vi "CameraTest.vi"() -> ()   [LabVIEW 2016]
uses:
  <vilib>/userdefined/High Color/IMAQdx.ctl
  ListboxMenu/listbox/listbox.lvclass
  ListboxMenu/listbox/listbox.lvclass/listbox.ctl
  ListboxMenu/LNK/UP/UP.lvclass
  C:/Users/ok/Desktop/camera parameters/ListboxMenu/LNK/Parent Class/Menu.lvclass
  ListboxMenu/LNK/Delete/Delete.lvclass
  ListboxMenu/LNK/Down/Down.lvclass
  <vilib>/Utility/miscctls.llb/LVRowAndColumnTypeDef.ctl
  <vilib>/Utility/miscctls.llb/LVPositionTypeDef.ctl
  <vilib>/vision/driver/NI_Vision_Acquisition_Software.lvlib
  <resource>/objmgr/imaqdx.rc
  <vilib>/ptbypt/NI_PtbyPt.lvlib
panel:
  in  "搜索相机":bool
  in  "启动相机":bool
  in  "停止相机":bool
  in  "连续获取":bool
  in  "单次获取":bool
  out "Image":T1(plugin-control)
  in  "Enum":u16(ring) items=["Off", "On"]
  in  "String":string
  in  "U32":i16
  in  "I64":i64
  in  "DBL":dbl
  in  "Bool":bool
  in  "写入参数文件":bool
  in  "读取参数文件":bool
  in  "相机参数列表":u16(ring) items=["NULL", "AcquisitionAttributes::AdvancedEthernet::BandwidthControl::DesiredPeakBandwidth", "AcquisitionAttributes::AdvancedEthernet::Controller::DestinationMode", "AcquisitionAttributes::AdvancedEthernet::Controller::DestinationMulticastAddress", "AcquisitionAttributes::AdvancedEthernet::EventParameters::MaxOutstandingEvents", "AcquisitionAttributes::AdvancedEthernet::FirewallTraversal::Enabled", "AcquisitionAttributes::AdvancedEthernet::FirewallTraversal::KeepAliveTime", "AcquisitionAttributes::AdvancedEthernet::ResendParameters::MaxResendsPerPacket", "AcquisitionAttributes::AdvancedEthernet::ResendParameters::MemoryWindowSize", "AcquisitionAttributes::AdvancedEthernet::ResendParameters::MissingPacketTimeout", "AcquisitionAttributes::AdvancedEthernet::ResendParameters::NewPacketTimeout", "AcquisitionAttributes::AdvancedEthernet::ResendParameters::ResendBatchingPercentage", "AcquisitionAttributes::AdvancedEthernet::ResendParameters::ResendResponseTimeout", "AcquisitionAttributes::AdvancedEthernet::ResendParameters::ResendThresholdPercentage", "AcquisitionAttributes::AdvancedEthernet::ResendParameters::ResendTimerResolution", "AcquisitionAttributes::AdvancedEthernet::ResendParameters::ResendsEnabled", "AcquisitionAttributes::AdvancedEthernet::TestPacketParameters::MaxTestPacketRetries", "AcquisitionAttributes::AdvancedEthernet::TestPacketParameters::TestPacketEnabled", "AcquisitionAttributes::AdvancedEthernet::TestPacketParameters::TestPacketTimeout", "AcquisitionAttributes::AdvancedGenicam::CommandTimeout", "AcquisitionAttributes::AdvancedGenicam::EventsEnabled", "AcquisitionAttributes::AdvancedGenicam::IgnoreCameraValidationErrors", "AcquisitionAttributes::Bayer::Algorithm", "AcquisitionAttributes::Bayer::GainB", "AcquisitionAttributes::Bayer::GainG", "AcquisitionAttributes::Bayer::GainR", "AcquisitionAttributes::Bayer::Pattern", "AcquisitionAttributes::ChunkDataDecoding::ChunkDataDecodingEnabled", "AcquisitionAttributes::ChunkDataDecoding::MaximumChunkCopySize", "CameraAttributes::AnalogControls::GainAuto", "CameraAttributes::AnalogControls::GainSelector", "CameraAttributes::AnalogControls::GainRaw", "CameraAttributes::AnalogControls::BlackLevelSelector", "CameraAttributes::AnalogControls::BlackLevelRaw", "CameraAttributes::AnalogControls::GammaEnable", "CameraAttributes::AnalogControls::GammaSelector", "CameraAttributes::AnalogControls::Gamma", "CameraAttributes::AnalogControls::DigitalShift", "CameraAttributes::ImageFormat::PixelFormat", "CameraAttributes::ImageFormat::ReverseX", "CameraAttributes::ImageFormat::TestImageSelector", "CameraAttributes::AOI::Width", "CameraAttributes::AOI::Height", "CameraAttributes::AOI::OffsetX", "CameraAttributes::AOI::OffsetY", "CameraAttributes::AOI::CenterX", "CameraAttributes::AOI::CenterY", "CameraAttributes::AOI::BinningHorizontal", "CameraAttributes::AOI::BinningVertical", "CameraAttributes::AcquisitionTrigger::AcquisitionMode", "CameraAttributes::AcquisitionTrigger::AcquisitionFrameCount", "CameraAttributes::AcquisitionTrigger::TriggerSelector", "CameraAttributes::AcquisitionTrigger::TriggerMode", "CameraAttributes::AcquisitionTrigger::TriggerSoftware", "CameraAttributes::AcquisitionTrigger::TriggerSource", "CameraAttributes::AcquisitionTrigger::TriggerActivation", "CameraAttributes::AcquisitionTrigger::TriggerDelayAbs", "CameraAttributes::AcquisitionTrigger::ExposureMode", "CameraAttributes::AcquisitionTrigger::ExposureAuto", "CameraAttributes::AcquisitionTrigger::ExposureTimeAbs", "CameraAttributes::AcquisitionTrigger::ExposureTimeRaw", "CameraAttributes::AcquisitionTrigger::GlobalResetReleaseModeEnable", "CameraAttributes::AcquisitionTrigger::AcquisitionFrameRateEnable", "CameraAttributes::AcquisitionTrigger::AcquisitionFrameRateAbs", "CameraAttributes::AcquisitionTrigger::AcquisitionStatusSelector", "CameraAttributes::DigitalIO::LineSelector", "CameraAttributes::DigitalIO::LineMode", "CameraAttributes::DigitalIO::LineFormat", "CameraAttributes::DigitalIO::LineSource", "CameraAttributes::DigitalIO::LineInverter", "CameraAttributes::DigitalIO::UserOutputSelector", "CameraAttributes::DigitalIO::UserOutputValue", "CameraAttributes::DigitalIO::UserOutputValueAll", "CameraAttributes::SequenceControl::SequenceEnable", "CameraAttributes::SequenceControl::SequenceControlConfiguration::SequenceAdvanceMode", "CameraAttributes::SequenceControl::SequenceSetTotalNumber", "CameraAttributes::SequenceControl::SequenceSetIndex", "CameraAttributes::SequenceControl::SequenceSetStore", "CameraAttributes::SequenceControl::SequenceSetLoad", "CameraAttributes::SequenceControl::SequenceSetExecutions", "CameraAttributes::TimerControls::TimerDelayTimebaseAbs", "CameraAttributes::TimerControls::TimerDurationTimebaseAbs", "CameraAttributes::TimerControls::TimerSelector", "CameraAttributes::TimerControls::TimerDelayAbs", "CameraAttributes::TimerControls::TimerDelayRaw", "CameraAttributes::TimerControls::TimerDurationAbs", "CameraAttributes::TimerControls::TimerDurationRaw", "CameraAttributes::TimerControls::TimerTriggerSource", "CameraAttributes::TimerControls::TimerTriggerActivation", "CameraAttributes::TimerControls::CounterSelector", "CameraAttributes::TimerControls::CounterEventSource", "CameraAttributes::TimerControls::CounterResetSource", "CameraAttributes::LUTControls::LUTSelector", "CameraAttributes::LUTControls::LUTEnable", "CameraAttributes::LUTControls::LUTIndex", "CameraAttributes::LUTControls::LUTValue", "CameraAttributes::UserDefinedValues::UserDefinedValueSelector", "CameraAttributes::UserDefinedValues::UserDefinedValue", "CameraAttributes::DeviceInformation::DeviceUserID", "CameraAttributes::ChunkDataStreams::ChunkModeActive", "CameraAttributes::EventsGeneration::EventSelector", "CameraAttributes::EventsGeneration::EventNotification", "CameraAttributes::UserSets::UserSetSelector", "CameraAttributes::UserSets::UserSetLoad", "CameraAttributes::UserSets::UserSetSave", "CameraAttributes::UserSets::UserSetDefaultSelector", "CameraAttributes::UserSets::DefaultSetSelector", "CameraAttributes::TransportLayer::GevSCFTD", "CameraAttributes::TransportLayer::GevSCBWR", "CameraAttributes::TransportLayer::GevSCBWRA", "CameraAttributes::TransportLayer::GevTimestampControlReset", "CameraAttributes::TransportLayer::GevTimestampControlLatchReset", "CameraAttributes::FileAccessControl::FileSelector", "CameraAttributes::FileAccessControl::FileOperationSelector", "CameraAttributes::FileAccessControl::FileOpenMode", "CameraAttributes::FileAccessControl::FileAccessOffset", "CameraAttributes::FileAccessControl::FileAccessLength", "CameraAttributes::FileAccessControl::FileOperationExecute", "CameraAttributes::AutoFunctions::AutoTargetValue", "CameraAttributes::AutoFunctions::AutoGainRawLowerLimit", "CameraAttributes::AutoFunctions::AutoGainRawUpperLimit", "CameraAttributes::AutoFunctions::AutoExposureTimeAbsLowerLimit", "CameraAttributes::AutoFunctions::AutoExposureTimeAbsUpperLimit", "CameraAttributes::AutoFunctions::AutoFunctionProfile", "CameraAttributes::AutoFunctions::AutoFunctionAOIs::AutoFunctionAOISelector", "CameraAttributes::AutoFunctions::AutoFunctionAOIs::AutoFunctionAOIWidth", "CameraAttributes::AutoFunctions::AutoFunctionAOIs::AutoFunctionAOIHeight", "CameraAttributes::AutoFunctions::AutoFunctionAOIs::AutoFunctionAOIOffsetX", "CameraAttributes::AutoFunctions::AutoFunctionAOIs::AutoFunctionAOIOffsetY", "CameraAttributes::AutoFunctions::AutoFunctionAOIs::AutoFunctionAOIUsageIntensity", "CameraAttributes::AutoFunctions::AutoFunctionAOIs::AutoFunctionAOIUsageWhiteBalance", "CameraAttributes::ExpertFeatureAccess::ExpertFeatureAccessSelector", "CameraAttributes::ExpertFeatureAccess::ExpertFeatureAccessKey", "AcquisitionAttributes::BitsPerPixel", "AcquisitionAttributes::ImageDecoderCopyMode", "AcquisitionAttributes::IncompleteBufferMode", "AcquisitionAttributes::OutputImageType", "AcquisitionAttributes::OverwriteMode", "AcquisitionAttributes::PacketSize", "AcquisitionAttributes::ReceiveTimestampMode", "AcquisitionAttributes::ShiftPixelBits", "AcquisitionAttributes::SwapPixelBytes", "AcquisitionAttributes::Timeout"]
  in  "添加参数":bool
  in  "写入参数":bool
  in  "获取参数值":bool
  in  "打开相机":bool
  in  "相机参数":i32(listbox)
  in  "相机列表":u16(ring) items=["acA2500-14gm:\"cam0\""]
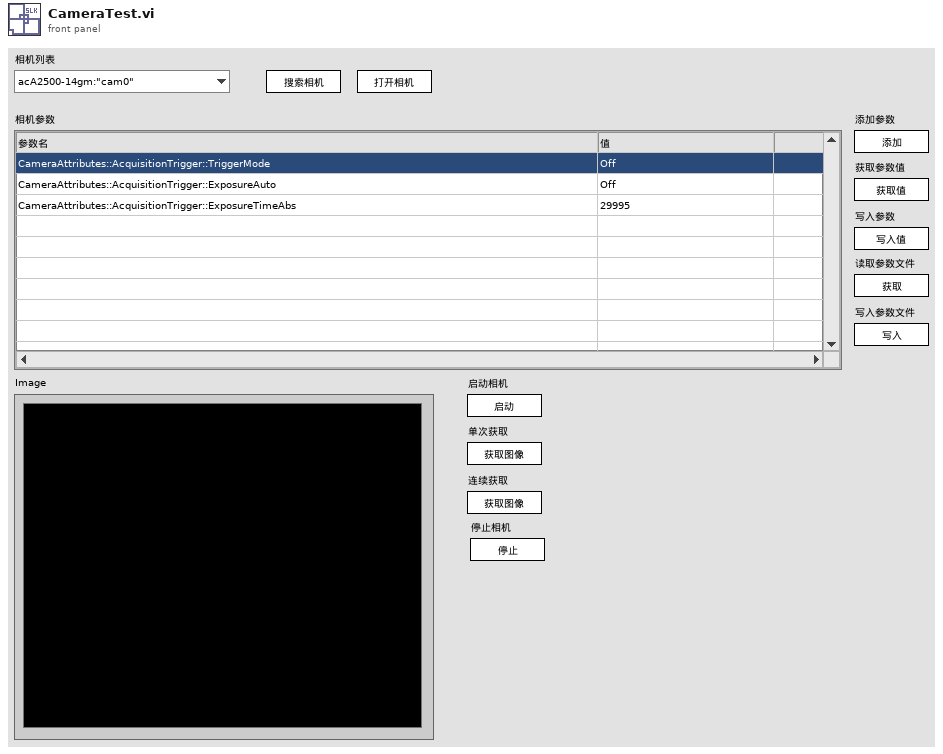
[diagram p1: front panel]
types:
  T1 = typedef "IMAQ Image.ctl" = refnum<image>
  T2 = typedef "Image Type" = u32
  T3 = typedef "IMAQdx.ctl" = refnum<k21>
  T4 = typedef "LVRowAndColumnTypeDef.ctl" = cluster{"Row":i32, "Column":i32}
  T5 = typedef "LVPositionTypeDef.ctl" = cluster{"Left":i32, "Top":i32}
  T6 = cluster{"Type":u32, "Version":u32, "Flags":u32, "SerialNumberHigh":u32, "SerialNumberLow":u32, "BusType":u32, "InterfaceName":string, "VendorName":string, "ModelName":string, "CameraFileName":string, "CameraAttributeURL":string}[]
  T7 = cluster{"Type":u32, "Version":u32, "Flags":u32, "SerialNumberHigh":u32, "SerialNumberLow":u32, "BusType":u32, "InterfaceName":string, "VendorName":string, "ModelName":string, "CameraFileName":string, "CameraAttributeURL":string}
  T8 = typedef "LVPoint32TypeDef.ctl" = cluster{"Horizontal":i32, "Vertical":i32}
  T9 = typedef "NI_Vision_Acquisition_Software.lvlib/IMAQdx Attribute Type.ctl" = enum32{"U32", "I64", "DBL", "String", "Enum", "Bool", "Command"}
  T10 = cluster{"Attribute Type":T9, "Readable":bool, "Writable":bool, "Attribute Name":string}[]
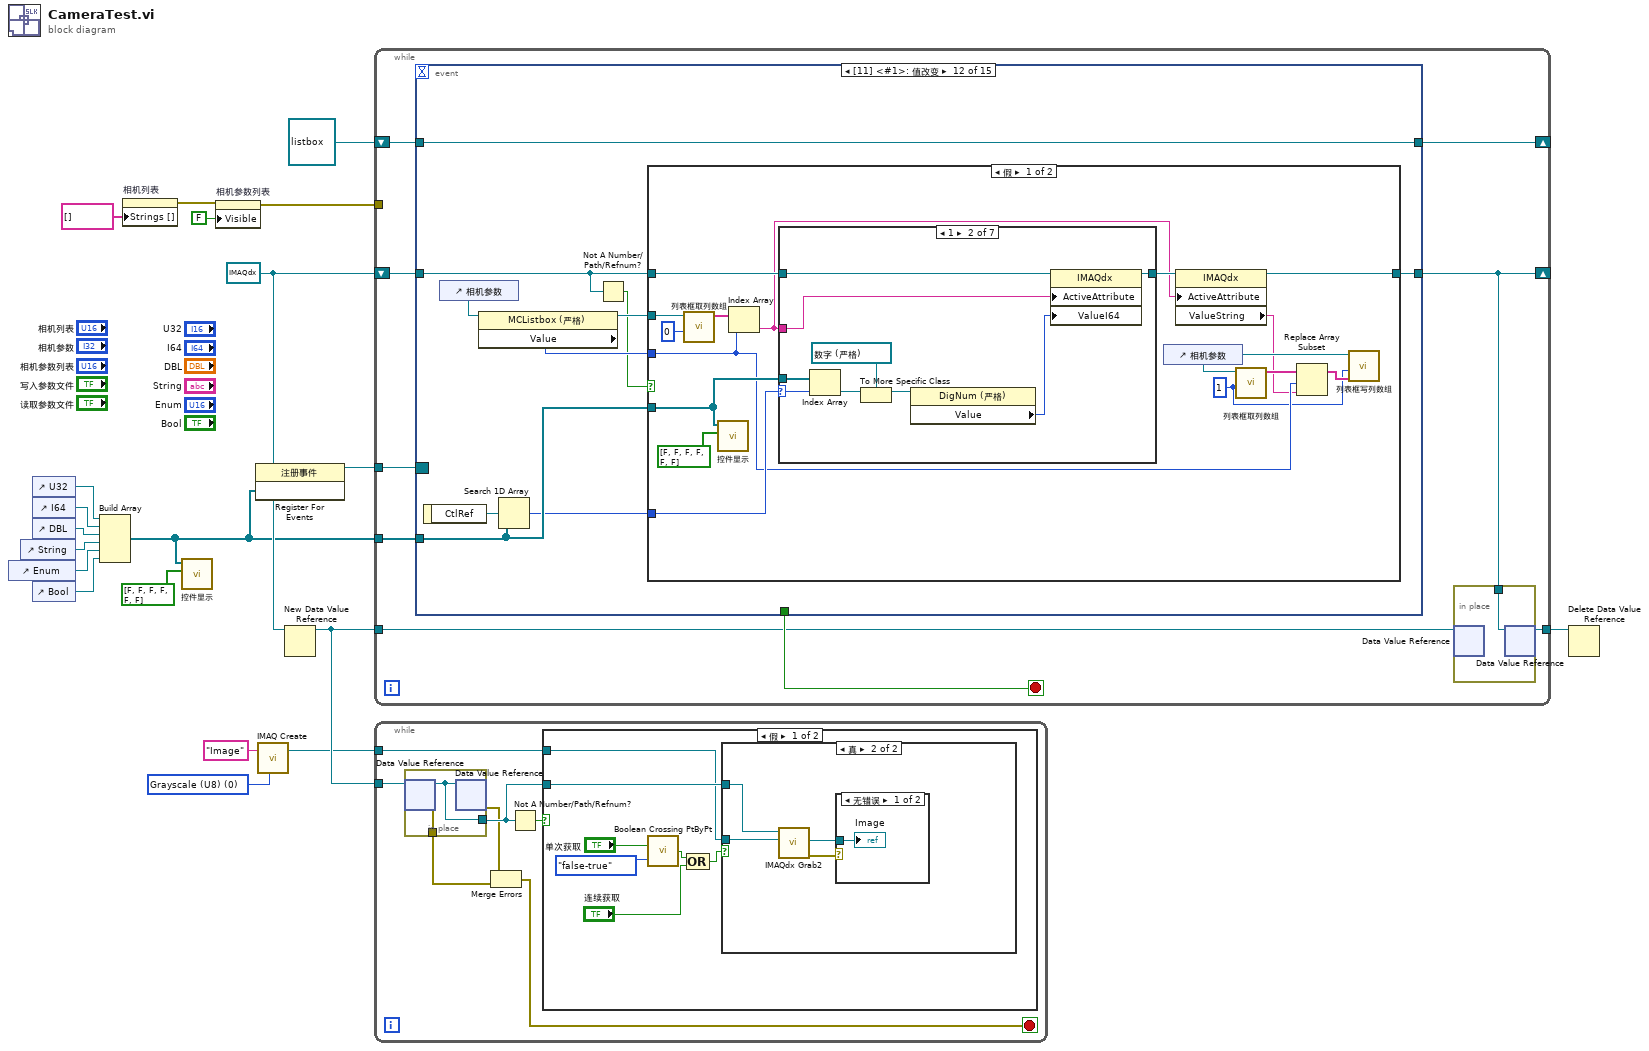
[diagram p0: block diagram]
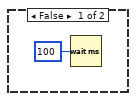
[diagram p2: hidden frame]
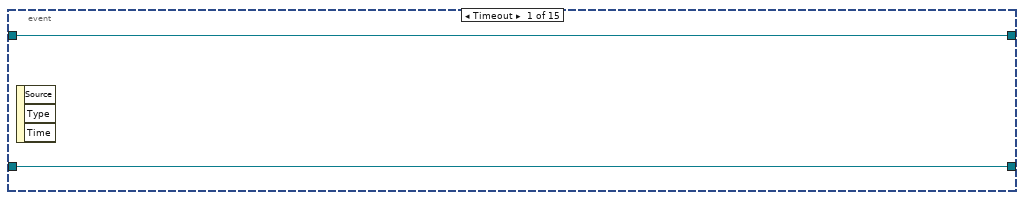
[diagram p5: hidden frame]
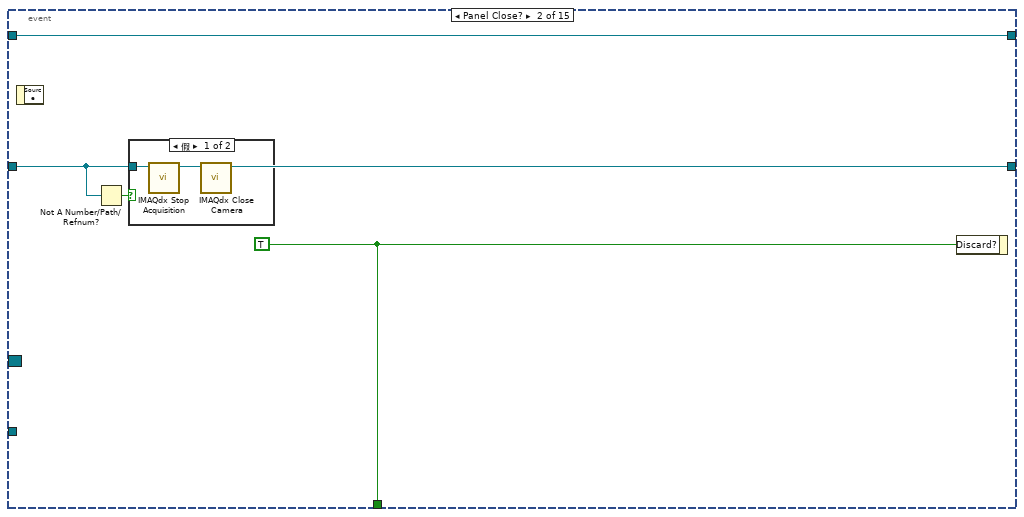
[diagram p6: hidden frame]
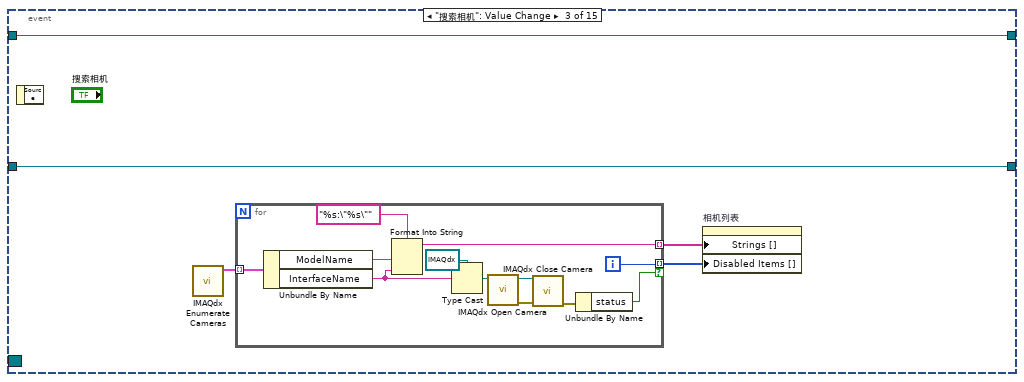
[diagram p8: hidden frame]
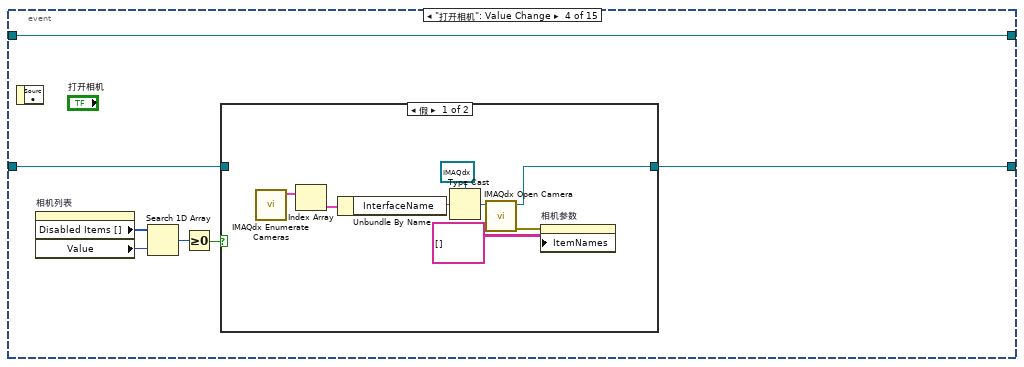
[diagram p9: hidden frame]
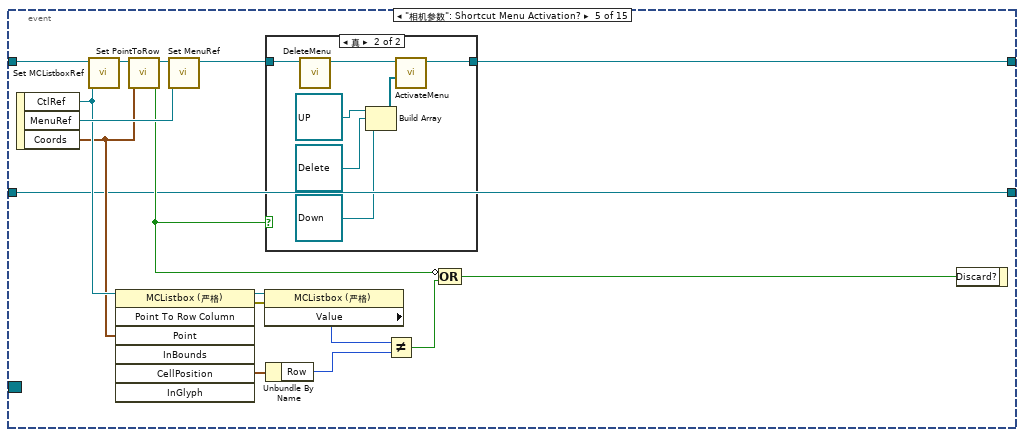
[diagram p11: hidden frame]
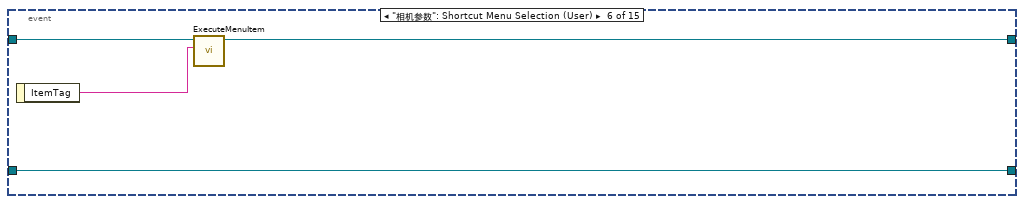
[diagram p13: hidden frame]
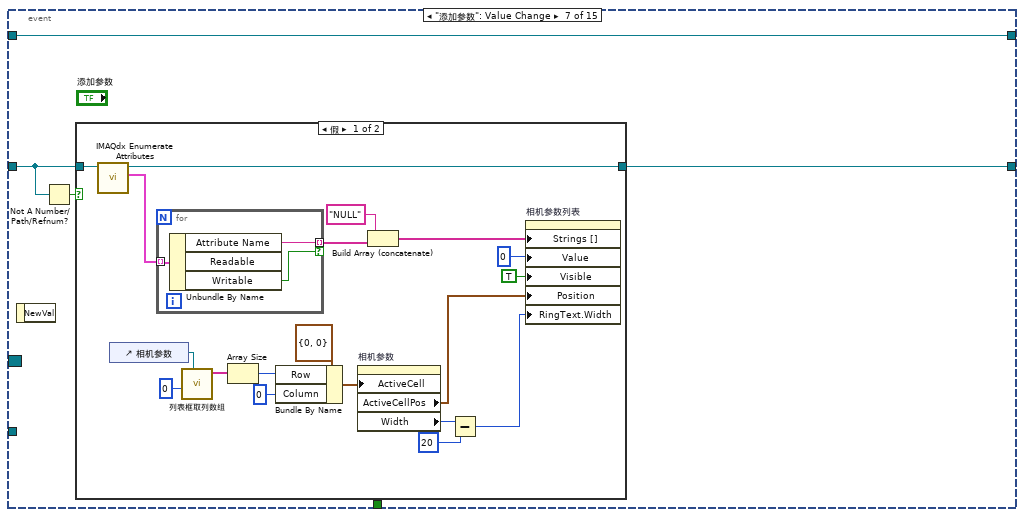
[diagram p14: hidden frame]
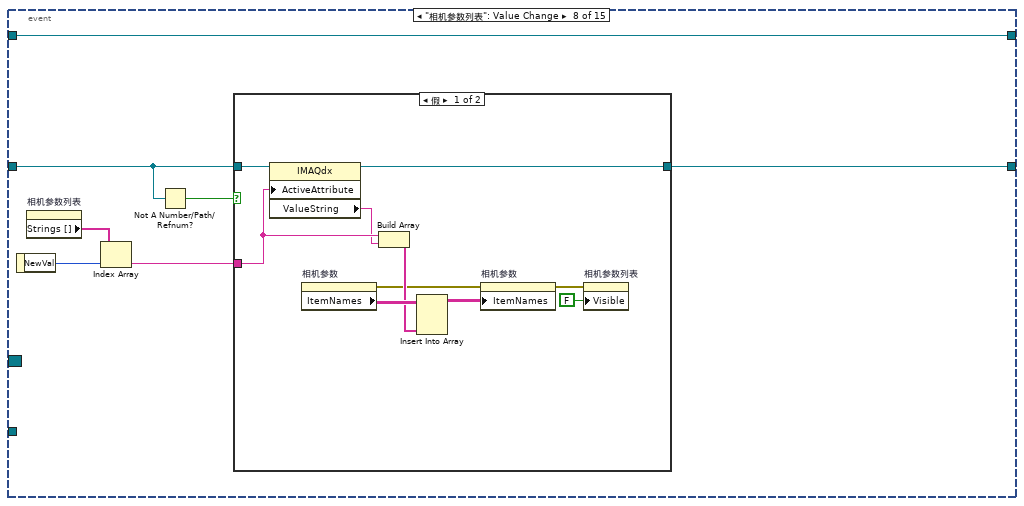
[diagram p16: hidden frame]
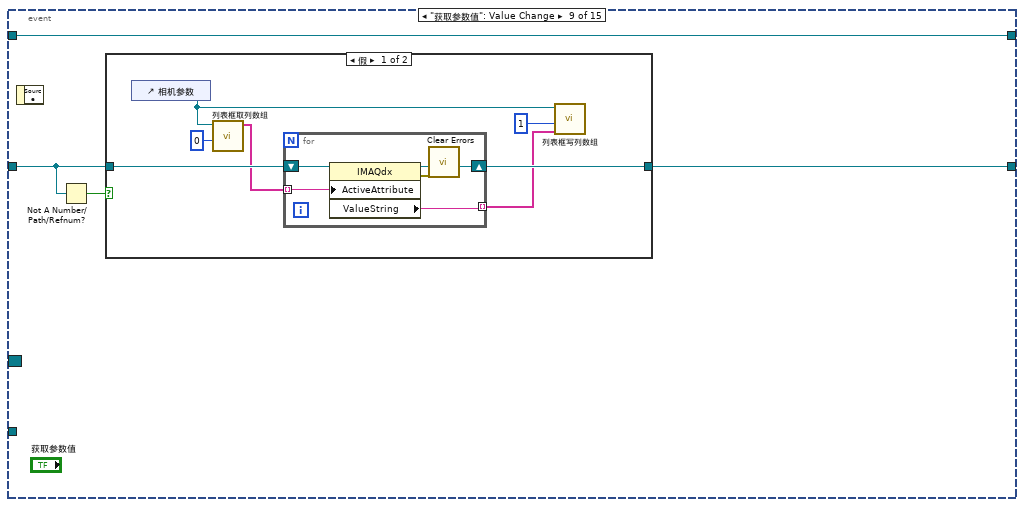
[diagram p18: hidden frame]
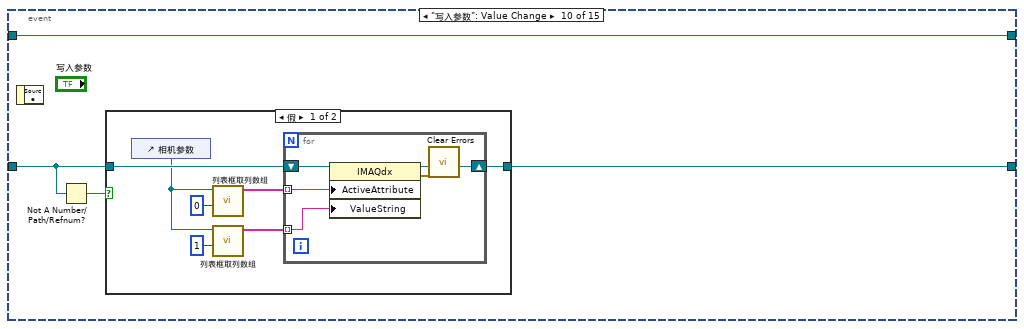
[diagram p20: hidden frame]
diagram:
  w4 = T2 0 items=["Grayscale (U8)", "Grayscale (I16)", "Grayscale (SGL)", "Complex (CSG)", "RGB (U32)", "HSL (U32)", "RGB (U64)", "Grayscale (U16)"] ("Image Type")
  w17 = T3 refnum ("Session In")
  n1 = control-ref of="Enum"() -> (w14:refnum<vi>)
  n2 = control-ref of="String"() -> (w11:refnum<vi>)
  n3 = control-ref of="U32"() -> (w16:refnum<vi>)
  n4 = control-ref of="I64"() -> (w13:refnum<vi>)
  n5 = control-ref of="DBL"() -> (w12:refnum<vi>)
  n6 = control-ref of="Bool"() -> (w15:refnum<vi>)
  n7 = Build Array(w16, w13, w12, w11, w14, w15) -> (w9:refnum<vi>[])
  n8 = property on="相机列表" class="Ring (严格)"("Strings []"=string[] [] ("字符串[]")) -> (error out=w1:errorcluster)  [unwired: 2 in, 1 out]
  n9 = call "控件显示.vi"("Visible"=bool[] [FALSE, FALSE, FALSE, FALSE, FALSE, FALSE], "Ctl"=w9) -> ()  [unwired: 10 in]
  n10 = property on="相机参数列表" class="Ring (严格)"(error in=w1, "Visible"=FALSE ("可见")) -> (error out=w18:errorcluster)  [unwired: 1 in, 1 out]
  n11 = register-events(w9) -> (reference out=w8:refnum<event-registration>)  [unwired: 2 in, 1 out]
  n12 = call "IMAQ Create"("Image Name"="Image", "Image Type"=w4) -> ("New Image"=w3:T1)  [unwired: 3 in, 1 out]
  n13 = New Data Value Reference(data value=w17) -> (data value reference=w6:refnum<data-value>)  [unwired: 1 in, 1 out]
  n14 = while {
    shift-right: [w22] -> _
    shift-left: w17 -> [w28]
    shift-right: [w26] -> _
    shift-left: refnum<class "listbox.lvclass"> refnum ("listbox.lvclass") -> [w27]
    tunnel: w18 -> [_]
    tunnel: w9 -> [w25]
    tunnel: w8 -> [w24]
    tunnel: w6 -> [w23]
    tunnel: [w21] -> w7
    stop <- w29 stop-if-true
    n15 = event shown="[11] <#1>: 值改变" {
      selector: w24 -> [_ _ _ _ _ _ _ _ _ _ _ _ _ _ _]
      dyn-events: _ -> [_ _ _ _ _ _ _ _ _ _ _ _ _ _ _]
      timeout: _ -> [_ _ _ _ _ _ _ _ _ _ _ _ _ _ _]
      tunnel: [_ w36 _ _ _ _ _ _ _ _ _ _ _ _ _] -> w29
      tunnel: w28 -> [w32 w34 w42 w58 w72 w97 w103 w131 w147 w164 w181 w289 w366 w369 w376]
      tunnel: [w32 w34 w42 w57 w72 w97 w102 w130 w146 w163 w180 w288 w366 w368 w375] -> w22
      tunnel: w27 -> [w31 w33 w43 w56 w88 w100 w101 w134 w149 w166 w197 w292 w365 w370 w377]
      tunnel: [w31 w33 w43 w56 w86 w99 w101 w134 w149 w166 w197 w292 w365 w370 w377] -> w26
      tunnel: w25 -> [_ _ _ _ _ _ _ _ _ _ w182 w286 _ _ _]
      event Timeout {
        n16 = event-data() -> ()  [unwired: 1 in, 3 out]
      }
      event Panel Close? {
        w36 = TRUE ("放弃？")
        n17 = event-data() -> ()  [unwired: 1 in, 1 out]
        n18 = Not A Number/Path/Refnum?(number/path/refnum=w34) -> (NaN/Path/Refnum?=w35:bool)
        n19 = case shown="假" w35 {
          tunnel: w34 -> [w38 _]
          frame False {
            n20 = call <vilib>:"IMAQdx Stop Acquisition.vi"("Session In"=w38) -> ("Session Out"=w37:T3)  [unwired: 9 in, 1 out]
            n21 = call <vilib>:"IMAQdx Close Camera.vi"("Session In"=w37) -> ()  [unwired: 10 in, 1 out]
          }
          frame True {
          }
        }
        n22 = event-data("Discard?"=w36) -> ()  [unwired: 1 in, 1 out]
      }
      event "搜索相机": Value Change {
        n23 = event-data() -> ()  [unwired: 1 in, 1 out]
        n24 = call <vilib>:"IMAQdx Enumerate Cameras.vi"() -> ("Camera Information Array"=w40:T6)  [unwired: 10 in, 1 out]
        n25 = for {
          tunnel: w40 -> [w55] mode=indexing
          tunnel: [w52] -> w39 mode=indexing
          tunnel: [w51] -> w41 mode=indexing if=w47
          i -> [w51]
          n26 = Unbundle By Name(w55) -> ("ModelName"=w54:string, "InterfaceName"=w48:string)
          n27 = Format Into String(format string="%s:\"%s\"" ("格式字符串"), w54, w48) -> (resulting string=w52:string)  [unwired: 2 in, 1 out]
          n28 = Type Cast(type=T3 refnum ("Session In"), x=w48) -> (*(type *) &x=w49:T3)
          n29 = call <vilib>:"IMAQdx Open Camera.vi"("Session In"=w49) -> ("error out"=w46:errorcluster, "Session Out"=w45:T3)  [unwired: 9 in]
          n30 = call <vilib>:"IMAQdx Close Camera.vi"("error in"=w46, "Session In"=w45) -> ("error out"=w44:errorcluster)  [unwired: 9 in]
          n31 = Unbundle By Name(w44) -> ("status"=w47:bool)
        }
        n32 = property on="相机列表" class="Ring (严格)"("Strings []"=w39, "Disabled Items []"=w41) -> ()  [unwired: 2 in, 2 out]
      }
      event "打开相机": Value Change {
        n33 = event-data() -> ()  [unwired: 1 in, 1 out]
        n34 = property on="相机列表" class="Ring (严格)"() -> ("Disabled Items []"=w62:i32[], "Value"=w60:u16)  [unwired: 2 in, 2 out]
        n35 = Search 1D Array(1D array=w62, element=w60) -> (index of element=w61:i32)  [unwired: 1 in]
        n36 = Greater Or Equal To 0?(x=w61) -> (x >= 0?=w59:bool)
        n37 = case shown="假" w59 {
          tunnel: w58 -> [_ w71]
          tunnel: [w65 w71] -> w57
          frame False {
            n38 = call <vilib>:"IMAQdx Enumerate Cameras.vi"() -> ("Camera Information Array"=w69:T6)  [unwired: 10 in, 1 out]
            n39 = Index Array(array=w69) -> (element=w70:T7)  [unwired: 1 in]
            n40 = Unbundle By Name(w70) -> ("InterfaceName"=w66:string)
            n41 = Type Cast(type=T3 refnum ("Session In"), x=w66) -> (*(type *) &x=w68:T3)
            n42 = call <vilib>:"IMAQdx Open Camera.vi"("Session In"=w68) -> ("error out"=w64:errorcluster, "Session Out"=w65:T3)  [unwired: 9 in]
            n43 = property on="相机参数" class="MCListbox (严格)"(error in=w64, "ItemNames"=string[][] [] ("项名")) -> ()  [unwired: 1 in, 2 out]
          }
          frame True {
          }
        }
      }
      event "相机参数": Shortcut Menu Activation? {
        n44 = event-data() -> ("CtlRef"=w82:refnum<vi>, "MenuRef"=w84:refnum<k9>, "Coords"=w81:T8)  [unwired: 1 in]
        n45 = call "Set MCListboxRef.vi"("MCListboxRef"=w82, "listbox in"=w88) -> ("listbox out"=w87:refnum<class "listbox.lvclass">)  [unwired: 9 in]
        n46 = invoke class="MCListbox (严格)" method="Point To Row Column"(reference=w82, "Point"=w81) -> (reference out=w79:refnum<vi>, error out=w78:errorcluster, "CellPosition"=w80:T4)  [unwired: 5 in, 4 out]
        n47 = call "Set PointToRow.vi"("坐标"=w81, "listbox 输入"=w87) -> ("边界内？"=w75:bool, "listbox 输出"=w85:refnum<class "listbox.lvclass">)  [unwired: 7 in, 1 out]
        n48 = call "Set MenuRef.vi"("MenuRef"=w84, "listbox in"=w85) -> ("listbox out"=w83:refnum<class "listbox.lvclass">)  [unwired: 9 in]
        n49 = property class="MCListbox (严格)"(reference=w79, error in=w78) -> ("Value"=w77:i32)  [unwired: 2 out]
        n50 = case shown="真" w75 {
          tunnel: w83 -> [w89 w91]
          tunnel: [w89 w92] -> w86
          frame False {
          }
          frame True {
            n51 = call "DeleteMenu.vi"("listbox 输入"=w91) -> ("listbox 输出"=w90:refnum<class "listbox.lvclass">)  [unwired: 9 in, 1 out]
            n52 = Build Array(refnum<class "UP.lvclass"> refnum ("UP.lvclass"), refnum<class "Delete.lvclass"> refnum ("Delete.lvclass"), refnum<class "Down.lvclass"> refnum ("Down.lvclass")) -> (w93:refnum<class "Menu.lvclass">[])
            n53 = call "ActivateMenu.vi"("MenuClassArray"=w93, "listbox 输入"=w90) -> ("listbox 输出"=w92:refnum<class "listbox.lvclass">)  [unwired: 8 in, 1 out]
          }
        }
        n54 = Unbundle By Name(w80) -> ("Row"=w76:i32)
        n55 = Not Equal?(x=w77, y=w76) -> (x != y?=w74:bool)
        n56 = Compound Arithmetic op=OR ("复合运算")(invert w75, w74) -> (w73:bool)
        n57 = event-data("Discard?"=w73) -> ()  [unwired: 1 in, 1 out]
      }
      event "相机参数": Shortcut Menu Selection (User) {
        n58 = event-data() -> ("ItemTag"=w98:string)  [unwired: 1 in]
        n59 = call "ExecuteMenuItem.vi"("项标识符"=w98, "listbox 输入"=w100) -> ("listbox 输出"=w99:refnum<class "listbox.lvclass">)  [unwired: 8 in, 1 out]
      }
      event "添加参数": Value Change {
        n60 = event-data() -> ()  [unwired: 1 in, 1 out]
        n61 = Not A Number/Path/Refnum?(number/path/refnum=w103) -> (NaN/Path/Refnum?=w104:bool)
        n62 = case shown="假" w104 {
          tunnel: w103 -> [w123 w127]
          tunnel: [w122 w127] -> w102
          frame False {
            n63 = call <vilib>:"IMAQdx Enumerate Attributes.vi"("Session In"=w123) -> ("Attribute Information Array"=w121:T10, "Session Out"=w122:T3)  [unwired: 8 in, 1 out]
            n64 = control-ref of="相机参数"() -> (w107:refnum<vi>)
            n65 = for {
              tunnel: w121 -> [w126] mode=indexing
              tunnel: [w125] -> w119 mode=indexing if=w124
              n66 = Unbundle By Name(w126) -> ("Attribute Name"=w125:string, "Writable"=w124:bool)  [unwired: 1 out]
            }
            n67 = call "列表框取列数组.vi"("列"=0, "引用"=w107) -> ("列数组"=w105:string[])  [unwired: 9 in]
            n68 = Array Size(array=w105) -> (size(s)=w114:i32)
            n69 = Bundle By Name(cluster=T4 {"Row"=0, "Column"=0} ("活动单元格:活动单元格"), "Row"=w114, "Column"=0) -> (w116:T4)
            n70 = property on="相机参数" class="MCListbox (严格)"("ActiveCell"=w116) -> ("ActiveCellPos"=w112:T5, "Width"=w111:u32)  [unwired: 2 in, 2 out]
            n71 = Build Array (concatenate)("NULL", w119) -> (w117:string[])
            n72 = Subtract(x=w111, y=u32 20) -> (x-y=w109:u32)
            n73 = property on="相机参数列表" class="Ring (严格)"("Strings []"=w117, "Value"=u16 0, "Visible"=TRUE ("可见"), "Position"=w112, "RingText.Width"=w109) -> ()  [unwired: 2 in, 2 out]
          }
          frame True {
          }
        }
      }
      event "相机参数列表": Value Change {
        n74 = event-data() -> ("NewVal"=w132:u16)  [unwired: 1 in]
        n75 = property on="相机参数列表" class="Ring (严格)"() -> ("Strings []"=w133:string[])  [unwired: 2 in, 2 out]
        n76 = Index Array(array=w133, index=w132) -> (element=w128:string)
        n77 = Not A Number/Path/Refnum?(number/path/refnum=w131) -> (NaN/Path/Refnum?=w129:bool)
        n78 = case shown="假" w129 {
          tunnel: w131 -> [w144 w145]
          tunnel: [w143 w145] -> w130
          tunnel: w128 -> [w142 _]
          frame False {
            n79 = property class="IMAQdx"(reference=w144, "ActiveAttribute"=w142) -> (reference out=w143:T3, "ValueString"=w141:string)  [unwired: 1 in, 1 out]
            n80 = property on="相机参数" class="MCListbox (严格)"() -> (error out=w137:errorcluster, "ItemNames"=w140:string[][])  [unwired: 2 in, 1 out]
            n81 = Build Array(w142, w141) -> (w139:string[])
            n82 = Insert Into Array(array=w140, new element=w139) -> (w138:string[][])  [unwired: 2 in]
            n83 = property on="相机参数" class="MCListbox (严格)"(error in=w137, "ItemNames"=w138) -> (error out=w136:errorcluster)  [unwired: 1 in, 1 out]
            n84 = property on="相机参数列表" class="Ring (严格)"(error in=w136, "Visible"=FALSE ("可见")) -> ()  [unwired: 1 in, 2 out]
          }
          frame True {
          }
        }
      }
      event "获取参数值": Value Change {
        n85 = event-data() -> ()  [unwired: 1 in, 1 out]
        n86 = Not A Number/Path/Refnum?(number/path/refnum=w147) -> (NaN/Path/Refnum?=w148:bool)
        n87 = case shown="假" w148 {
          tunnel: w147 -> [w155 w162]
          tunnel: [w154 w162] -> w146
          frame False {
            n88 = control-ref of="相机参数"() -> (w152:refnum<vi>)
            n89 = call "列表框取列数组.vi"("列"=0, "引用"=w152) -> ("列数组"=w153:string[])  [unwired: 9 in]
            n90 = for {
              shift-right: [w160] -> w154
              shift-left: w155 -> [w161]
              tunnel: w153 -> [w159] mode=indexing
              tunnel: [w158] -> w150 mode=indexing
              n91 = property class="IMAQdx"(reference=w161, "ActiveAttribute"=w159) -> (reference out=w160:T3, error out=w157:errorcluster, "ValueString"=w158:string)  [unwired: 1 in]
              n92 = call <vilib>:"Clear Errors.vi"("error in (no error)"=w157) -> ()  [unwired: 5 in, 2 out]
            }
            n93 = call "列表框写列数组.vi"("新元素/子数组"=w150, "列"=1, "引用"=w152) -> ()  [unwired: 9 in]
          }
          frame True {
          }
        }
      }
      event "写入参数": Value Change {
        n94 = event-data() -> ()  [unwired: 1 in, 1 out]
        n95 = Not A Number/Path/Refnum?(number/path/refnum=w164) -> (NaN/Path/Refnum?=w165:bool)
        n96 = case shown="假" w165 {
          tunnel: w164 -> [w172 w179]
          tunnel: [w171 w179] -> w163
          frame False {
            n97 = control-ref of="相机参数"() -> (w168:refnum<vi>)
            n98 = call "列表框取列数组.vi"("列"=0, "引用"=w168) -> ("列数组"=w170:string[])  [unwired: 9 in]
            n99 = call "列表框取列数组.vi"("列"=1, "引用"=w168) -> ("列数组"=w167:string[])  [unwired: 9 in]
            n100 = for {
              shift-right: [w177] -> w171
              shift-left: w172 -> [w178]
              tunnel: w170 -> [w176] mode=indexing
              tunnel: w167 -> [w174] mode=indexing
              n101 = property class="IMAQdx"(reference=w178, "ActiveAttribute"=w176, "ValueString"=w174) -> (reference out=w177:T3, error out=w175:errorcluster)  [unwired: 1 in]
              n102 = call <vilib>:"Clear Errors.vi"("error in (no error)"=w175) -> ()  [unwired: 5 in, 2 out]
            }
          }
          frame True {
          }
        }
      }
      event "相机参数": Mouse Down {
        n103 = event-data() -> ("CtlRef"=w192:refnum<vi>, "Coords"=w191:T8)  [unwired: 1 in]
        n104 = invoke class="MCListbox (严格)" method="Point To Row Column"(reference=w192, "Point"=w191) -> (reference out=w195:refnum<vi>, error out=w194:errorcluster, "CellPosition"=w196:T4)  [unwired: 5 in, 4 out]
        n105 = property class="MCListbox (严格)"(reference=w195, error in=w194) -> (reference out=w188:refnum<vi>, "Value"=w187:i32)  [unwired: 1 out]
        n106 = Unbundle By Name(w196) -> ("Row"=w193:i32, "Column"=w190:i32)
        n107 = Equal?(x=w187, y=w193) -> (x = y?=w185:bool)
        n108 = Equal?(x=w190, y=1) -> (x = y?=w184:bool)
        n109 = Not A Number/Path/Refnum?(number/path/refnum=w181) -> (NaN/Path/Refnum?=w186:bool)
        n110 = Compound Arithmetic op=AND ("复合运算")(invert w186, w185, w184) -> (w183:bool)
        n111 = case shown="真" w183 {
          tunnel: w188 -> [_ w209]
          tunnel: w187 -> [_ w208]
          tunnel: w181 -> [w198 w212]
          tunnel: w182 -> [_ w201]
          tunnel: [w198 w199] -> w180
          frame False {
          }
          frame True {
            n112 = Bundle By Name(cluster=T4 {"Row"=0, "Column"=0} ("活动单元格:活动单元格"), "Row"=w208, "Column"=1) -> (w211:T4)
            n113 = call "列表框取列数组.vi"("列"=0, "引用"=w209) -> ("列数组"=w213:string[])  [unwired: 9 in]
            n114 = Index Array(array=w213, index=w208) -> (element=w202:string)
            n115 = property on="属性节点" class="MCListbox (严格)"(reference=w209, "ActiveCell"=w211) -> ("ActiveCellPos"=w206:T5)  [unwired: 1 in, 2 out]
            n116 = property class="IMAQdx"(reference=w212, "ActiveAttribute"=w202) -> (reference out=w203:T3, "Type"=w204:u32)  [unwired: 1 in, 1 out]
            n117 = Add(x=w206, y=T5 {"Left"=50, "Top"=0}) -> (x+y=w200:T5)
            n118 = case shown="5" w204 {
              selector: w204 -> [w223 w234 w245 w256 w268 w279 _]
              tunnel: w203 -> [w225 w236 w247 w258 w270 w281 w282]
              tunnel: w202 -> [w224 w235 w246 w257 w269 w280 _]
              tunnel: w201 -> [w216 w227 w239 w251 w264 w275 _]
              tunnel: w200 -> [w218 w231 w242 w253 w265 w276 _]
              tunnel: [w215 w226 w237 w248 w259 w271 w282] -> w199
              frame 0 {
                n119 = property class="IMAQdx"(reference=w225, "ActiveAttribute"=w224) -> (reference out=w215:T3, "ValueU32"=w220:u32)  [unwired: 1 in, 1 out]
                n120 = Index Array(array=w216, index=w223) -> (element=w222:refnum<vi>)
                n121 = To More Specific Class(target class=refnum<vi> refnum ("U32"), reference=w222) -> (specific class reference=w219:refnum<vi>)  [unwired: 1 in, 1 out]
                n122 = property class="DigNum (严格)"(reference=w219, "Value"=w220, "Position"=w218) -> ()  [unwired: 1 in, 2 out]
                n123 = call "控件显示.vi"("Visible"=bool[] [TRUE, FALSE, FALSE, FALSE, FALSE, FALSE], "Ctl"=w216) -> ()  [unwired: 10 in]
              }
              frame 1 {
                n124 = property class="IMAQdx"(reference=w236, "ActiveAttribute"=w235) -> (reference out=w226:T3, "ValueI64"=w229:i64)  [unwired: 1 in, 1 out]
                n125 = Index Array(array=w227, index=w234) -> (element=w233:refnum<vi>)
                n126 = To More Specific Class(target class=refnum<vi> refnum ("I64"), reference=w233) -> (specific class reference=w232:refnum<vi>)  [unwired: 1 in, 1 out]
                n127 = property class="DigNum (严格)"(reference=w232, "Value"=w229, "Position"=w231) -> ()  [unwired: 1 in, 2 out]
                n128 = call "控件显示.vi"("Visible"=bool[] [FALSE, TRUE, FALSE, FALSE, FALSE, FALSE], "Ctl"=w227) -> ()  [unwired: 10 in]
              }
              frame 2 {
                n129 = property class="IMAQdx"(reference=w247, "ActiveAttribute"=w246) -> (reference out=w237:T3, "ValueDBL"=w241:dbl)  [unwired: 1 in, 1 out]
                n130 = Index Array(array=w239, index=w245) -> (element=w244:refnum<vi>)
                n131 = To More Specific Class(target class=refnum<vi> refnum ("DBL"), reference=w244) -> (specific class reference=w243:refnum<vi>)  [unwired: 1 in, 1 out]
                n132 = property class="DigNum (严格)"(reference=w243, "Value"=w241, "Position"=w242) -> ()  [unwired: 1 in, 2 out]
                n133 = call "控件显示.vi"("Visible"=bool[] [FALSE, FALSE, TRUE, FALSE, FALSE, FALSE], "Ctl"=w239) -> ()  [unwired: 10 in]
              }
              frame 3 {
                n134 = property class="IMAQdx"(reference=w258, "ActiveAttribute"=w257) -> (reference out=w248:T3, "ValueString"=w252:string)  [unwired: 1 in, 1 out]
                n135 = Index Array(array=w251, index=w256) -> (element=w255:refnum<vi>)
                n136 = To More Specific Class(target class=refnum<vi> refnum ("String"), reference=w255) -> (specific class reference=w254:refnum<vi>)  [unwired: 1 in, 1 out]
                n137 = property class="Str"(reference=w254, "Value"=w252, "Position"=w253) -> ()  [unwired: 1 in, 2 out]
                n138 = call "控件显示.vi"("Visible"=bool[] [FALSE, FALSE, FALSE, TRUE, FALSE, FALSE], "Ctl"=w251) -> ()  [unwired: 10 in]
              }
              frame 4 {
                n139 = property class="IMAQdx"(reference=w270, "ActiveAttribute"=w269) -> (reference out=w259:T3, "EnumStrings[]"=w261:string[], "ValueU32"=w260:u32)  [unwired: 1 in, 1 out]
                n140 = Index Array(array=w264, index=w268) -> (element=w267:refnum<vi>)
                n141 = To More Specific Class(target class=refnum<vi> refnum ("Enum"), reference=w267) -> (specific class reference=w266:refnum<vi>)  [unwired: 1 in, 1 out]
                n142 = property class="Ring (严格)"(reference=w266, "Strings []"=w261, "Position"=w265, "Value"=w260) -> ()  [unwired: 1 in, 2 out]
                n143 = call "控件显示.vi"("Visible"=bool[] [FALSE, FALSE, FALSE, FALSE, TRUE, FALSE], "Ctl"=w264) -> ()  [unwired: 10 in]
              }
              frame 5 {
                n144 = property class="IMAQdx"(reference=w281, "ActiveAttribute"=w280) -> (reference out=w271:T3, "ValueBool"=w272:bool)  [unwired: 1 in, 1 out]
                n145 = Index Array(array=w275, index=w279) -> (element=w278:refnum<vi>)
                n146 = To More Specific Class(target class=refnum<vi> refnum ("Bool"), reference=w278) -> (specific class reference=w277:refnum<vi>)  [unwired: 1 in, 1 out]
                n147 = property class="Bool (严格)"(reference=w277, "Value"=w272, "Position"=w276) -> ()  [unwired: 1 in, 2 out]
                n148 = call "控件显示.vi"("Visible"=bool[] [FALSE, FALSE, FALSE, FALSE, FALSE, TRUE], "Ctl"=w275) -> ()  [unwired: 10 in]
              }
              frame 6, Default {
              }
            }
          }
        }
      }
      event Value Change {
        n149 = event-data() -> ("CtlRef"=w285:refnum<vi>)  [unwired: 1 in]
        n150 = control-ref of="相机参数"() -> (w287:refnum<vi>)
        n151 = property class="MCListbox (严格)"(reference=w287) -> (reference out=w291:refnum<vi>, "Value"=w290:i32)  [unwired: 1 in, 1 out]
        n152 = Search 1D Array(1D array=w286, element=w285) -> (index of element=w284:i32)  [unwired: 1 in]
        n153 = Not A Number/Path/Refnum?(number/path/refnum=w289) -> (NaN/Path/Refnum?=w283:bool)
        n154 = case shown="假" w283 {
          tunnel: w291 -> [w305 _]
          tunnel: w290 -> [w297 _]
          tunnel: w289 -> [w306 w364]
          tunnel: w286 -> [w302 _]
          tunnel: [w300 w364] -> w288
          tunnel: w284 -> [w304 _]
          frame False {
            w294 = 1 ("列")
            n155 = call "列表框取列数组.vi"("列"=0, "引用"=w305) -> ("列数组"=w307:string[])  [unwired: 9 in]
            n156 = call "控件显示.vi"("Visible"=bool[] [FALSE, FALSE, FALSE, FALSE, FALSE, FALSE], "Ctl"=w302) -> ()  [unwired: 10 in]
            n157 = Index Array(array=w307, index=w297) -> (element=w299:string)
            n158 = case shown="1" w304 {
              selector: w304 -> [w316 w325 w334 w343 w352 w361 _]
              tunnel: w306 -> [w311 w321 w330 w339 w348 w357 w363]
              tunnel: w299 -> [w317 w326 w335 w344 w353 w362 _]
              tunnel: w302 -> [w312 w322 w331 w340 w349 w358 _]
              tunnel: [w310 w320 w329 w338 w347 w356 w363] -> w301
              frame 0 {
                n159 = Index Array(array=w312, index=w316) -> (element=w315:refnum<vi>)
                n160 = To More Specific Class(target class=refnum<vi> refnum ("U32"), reference=w315) -> (specific class reference=w313:refnum<vi>)  [unwired: 1 in, 1 out]
                n161 = property class="DigNum (严格)"(reference=w313) -> ("Value"=w309:i16)  [unwired: 1 in, 2 out]
                n162 = property class="IMAQdx"(reference=w311, "ActiveAttribute"=w317, "ValueU32"=w309) -> (reference out=w310:T3)  [unwired: 1 in, 1 out]
              }
              frame 1 {
                n163 = Index Array(array=w322, index=w325) -> (element=w324:refnum<vi>)
                n164 = To More Specific Class(target class=refnum<vi> refnum ("I64"), reference=w324) -> (specific class reference=w323:refnum<vi>)  [unwired: 1 in, 1 out]
                n165 = property class="DigNum (严格)"(reference=w323) -> ("Value"=w319:i64)  [unwired: 1 in, 2 out]
                n166 = property class="IMAQdx"(reference=w321, "ActiveAttribute"=w326, "ValueI64"=w319) -> (reference out=w320:T3)  [unwired: 1 in, 1 out]
              }
              frame 2 {
                n167 = Index Array(array=w331, index=w334) -> (element=w333:refnum<vi>)
                n168 = To More Specific Class(target class=refnum<vi> refnum ("DBL"), reference=w333) -> (specific class reference=w332:refnum<vi>)  [unwired: 1 in, 1 out]
                n169 = property class="DigNum (严格)"(reference=w332) -> ("Value"=w328:dbl)  [unwired: 1 in, 2 out]
                n170 = property class="IMAQdx"(reference=w330, "ActiveAttribute"=w335, "ValueDBL"=w328) -> (reference out=w329:T3)  [unwired: 1 in, 1 out]
              }
              frame 3 {
                n171 = Index Array(array=w340, index=w343) -> (element=w342:refnum<vi>)
                n172 = To More Specific Class(target class=refnum<vi> refnum ("String"), reference=w342) -> (specific class reference=w341:refnum<vi>)  [unwired: 1 in, 1 out]
                n173 = property class="Str"(reference=w341) -> ("Value"=w337:string)  [unwired: 1 in, 2 out]
                n174 = property class="IMAQdx"(reference=w339, "ActiveAttribute"=w344, "ValueString"=w337) -> (reference out=w338:T3)  [unwired: 1 in, 1 out]
              }
              frame 4 {
                n175 = Index Array(array=w349, index=w352) -> (element=w351:refnum<vi>)
                n176 = To More Specific Class(target class=refnum<vi> refnum ("Enum"), reference=w351) -> (specific class reference=w350:refnum<vi>)  [unwired: 1 in, 1 out]
                n177 = property class="Ring (严格)"(reference=w350) -> ("Value"=w346:u16)  [unwired: 1 in, 2 out]
                n178 = property class="IMAQdx"(reference=w348, "ActiveAttribute"=w353, "ValueU32"=w346) -> (reference out=w347:T3)  [unwired: 1 in, 1 out]
              }
              frame 5 {
                n179 = Index Array(array=w358, index=w361) -> (element=w360:refnum<vi>)
                n180 = To More Specific Class(target class=refnum<vi> refnum ("Bool"), reference=w360) -> (specific class reference=w359:refnum<vi>)  [unwired: 1 in, 1 out]
                n181 = property class="Bool (严格)"(reference=w359) -> ("Value"=w355:bool)  [unwired: 1 in, 2 out]
                n182 = property class="IMAQdx"(reference=w357, "ActiveAttribute"=w362, "ValueBool"=w355) -> (reference out=w356:T3)  [unwired: 1 in, 1 out]
              }
              frame 6, Default {
              }
            }
            n183 = control-ref of="相机参数"() -> (w296:refnum<vi>)
            n184 = property class="IMAQdx"(reference=w301, "ActiveAttribute"=w299) -> (reference out=w300:T3, "ValueString"=w293:string)  [unwired: 1 in, 1 out]
            n185 = call "列表框取列数组.vi"("列"=w294, "引用"=w296) -> ("列数组"=w298:string[])  [unwired: 9 in]
            n186 = Replace Array Subset(array=w298, new element=w293, index=w297) -> (w295:string[])
            n187 = call "列表框写列数组.vi"("新元素/子数组"=w295, "列"=w294, "引用"=w296) -> ()  [unwired: 9 in]
          }
          frame True {
          }
        }
      }
      event "相机参数": Value Change {
        n188 = event-data() -> ()  [unwired: 1 in, 6 out]
      }
      event "启动相机": Value Change {
        n189 = event-data() -> ()  [unwired: 1 in, 6 out]
        n190 = Not A Number/Path/Refnum?(number/path/refnum=w369) -> (NaN/Path/Refnum?=w367:bool)
        n191 = case shown="假" w367 {
          tunnel: w369 -> [w372 w373]
          tunnel: [w371 w373] -> w368
          frame False {
            n192 = call <vilib>:"IMAQdx Configure Grab.vi"("Session In"=w372) -> ("Session Out"=w371:T3)  [unwired: 9 in, 1 out]
          }
          frame True {
          }
        }
      }
      event "停止相机": Value Change {
        n193 = event-data() -> ()  [unwired: 1 in, 6 out]
        n194 = Not A Number/Path/Refnum?(number/path/refnum=w376) -> (NaN/Path/Refnum?=w374:bool)
        n195 = case shown="假" w374 {
          tunnel: w376 -> [w380 w381]
          tunnel: [w379 w381] -> w375
          frame False {
            n196 = call <vilib>:"IMAQdx Stop Acquisition.vi"("Session In"=w380) -> ("Session Out"=w379:T3)  [unwired: 9 in, 1 out]
            n197 = local write "连续获取"(FALSE ("连续获取")) -> ()
          }
          frame True {
          }
        }
      }
    }
    n198 = in-place {
      in-place-border: w22 -> [w30]
      n199 = in-place-dvr #1(w23) -> ()  [unwired: 2 out]
      n200 = in-place-dvr #1(w30) -> (w21:refnum<data-value>)  [unwired: 1 out]
    }
  }
  n201 = while {
    tunnel: w6 -> [w388]
    tunnel: w3 -> [w385]
    stop <- w382 stop-if-true
    n202 = in-place {
      in-place-border: [w403] -> w386
      in-place-border: [w402] -> w383
      n203 = in-place-dvr #2(w388) -> (w403:T3, w402:errorcluster)
      n204 = in-place-dvr #2(w403) -> (w384:errorcluster)  [unwired: 1 out]
    }
    n205 = Merge Errors(w384, w383) -> (w382:errorcluster)
    n206 = Not A Number/Path/Refnum?(number/path/refnum=w386) -> (NaN/Path/Refnum?=w387:bool)
    n207 = case shown="假" w387 {
      tunnel: w386 -> [w393 _]
      tunnel: w385 -> [w392 _]
      frame False {
        n208 = call <vilib>:"Boolean Crossing PtByPt.vi"("direction"=enum16{"either", "false-true", "true-false"}."false-true", "input"="单次获取") -> ("crossing"=w391:bool)  [unwired: 1 in]
        n209 = Compound Arithmetic op=OR ("复合运算")(w391, "连续获取") -> (w389:bool)
        n210 = case shown="真" w389 {
          tunnel: w393 -> [_ w400]
          tunnel: w392 -> [_ w399]
          frame False {
            n211 = Wait (ms)(milliseconds to wait=u32 100 ("等待时间（毫秒）")) -> ()  [unwired: 1 out]
          }
          frame True {
            n212 = call <vilib>:"IMAQdx Grab2.vi"("Image In"=w399, "Session In"=w400) -> ("error out"=w397:errorcluster, "Image Out"=w398:T1)  [unwired: 6 in, 2 out]
            n213 = case shown="无错误" w397 {
              tunnel: w398 -> [w401 _]
              frame No Error {
                "Image" <- w401
              }
              frame Error {
              }
            }
          }
        }
      }
      frame True {
      }
    }
  }
  n214 = Delete Data Value Reference(data value reference=w7) -> ()  [unwired: 1 in, 2 out]
